vi "Untitled 3.vi"() -> ()   [LabVIEW 2016]
panel:
  in  "stop":bool
  out "Waveform Graph":dynamicdata(graph)
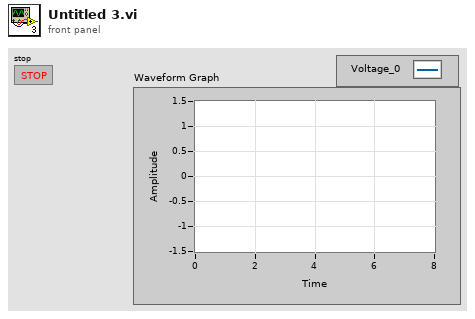
[diagram p1: front panel]
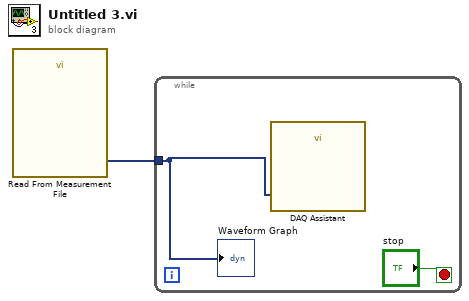
[diagram p0: block diagram]
diagram:
  n1 = call "Read From Measurement File"() -> ("Signals"=w1:dynamicdata)  [unwired: 6 in, 5 out]
  n2 = while {
    tunnel: w1 -> [w2]
    stop <- "stop" stop-if-true
    n3 = call "DAQ Assistant"("data"=w2) -> ()  [unwired: 17 in, 2 out]
    "Waveform Graph" <- w2
  }
